vi "LP Optimal FIR Filter.vi"(1 "Band Parameters":T1(array[cluster]), 2 "# of taps":i32) -> (0 "h new":dbl[](array[numeric]))   [LabVIEW 2023]
doc: "LP Optimal FIR Filter."
uses:
  <vilib>/Analysis/1siggen.llb/Ramp Pattern by Samples.vi
  <vilib>/Analysis/NI_AALBase.lvlib
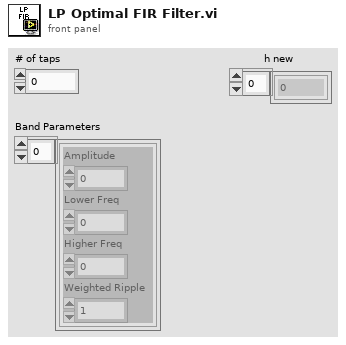
[diagram p1: front panel]
types:
  T1 = cluster{"Amplitude":dbl, "Lower Freq":dbl, "Higher Freq":dbl, "Weighted Ripple":dbl}[]
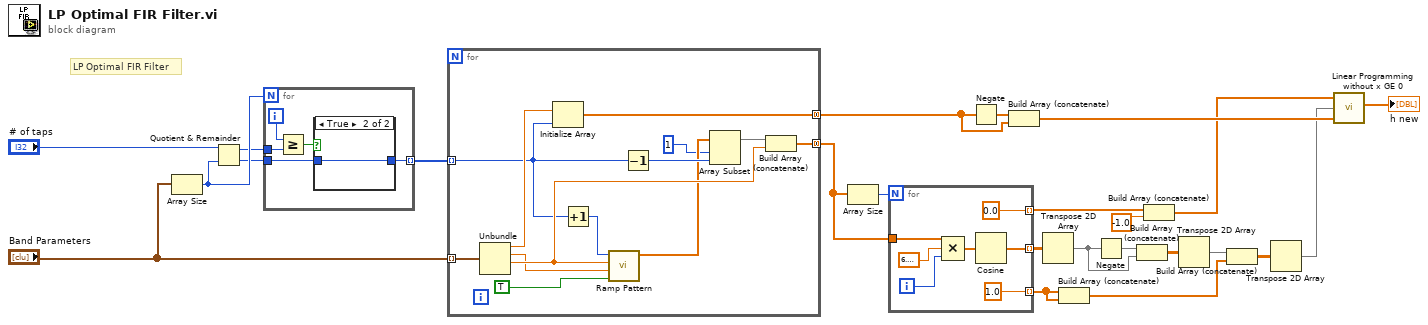
[diagram p0: block diagram]
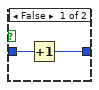
[diagram p2: hidden frame]
diagram:
  # "LP Optimal FIR Filter"
  n1 = Array Size(array="Band Parameters") -> (size(s)=w24:i32)
  n2 = Quotient & Remainder(x="# of taps", y=w24) -> (x-y*floor(x/y)=w23:i32, floor(x/y)=w22:i32)
  n3 = for {
    N: w24 -> [_]
    tunnel: w23 -> [w29]
    tunnel: w22 -> [w26]
    tunnel: [w25] -> w21 mode=indexing
    i -> [w28]
    n4 = Greater Or Equal?(x=w28, y=w29) -> (x >= y?=w27:bool)
    n5 = case shown="True" w27 {
      tunnel: w26 -> [w31 w32]
      tunnel: [w30 w32] -> w25
      frame False {
        n6 = Increment(x=w31) -> (x+1=w30:i32)
      }
      frame True {
      }
    }
  }
  n7 = for {
    tunnel: "Band Parameters" -> [w45] mode=indexing
    tunnel: w21 -> [w36] mode=indexing
    tunnel: [w35] -> w4 mode=concatenating
    tunnel: [w38] -> w2 mode=concatenating
    n8 = Unbundle(w45) -> ("Amplitude"=w37:dbl, "Lower Freq"=w34:dbl, "Higher Freq"=w41:dbl)  [unwired: 1 out]
    n9 = Initialize Array(w37, w36) -> (w35:dbl[])
    n10 = Increment(x=w36) -> (x+1=w42:i32)
    n11 = call-poly <vilib>:"Ramp Pattern.vi"("exclude end?"=TRUE, "start"=w34, "end"=w41, "samples"=w42) -> ("Ramp Pattern"=w39:dbl[])  [unwired: 6 in, 1 out]
    n12 = Decrement(x=w36) -> (x-1=w44:i32)
    n13 = Array Subset(array=w39, index=1, length=w44) -> (w43:dbl[])
    n14 = Build Array (concatenate)(w43, w41) -> (w38:dbl[])
  }
  n15 = Array Size(array=w2) -> (size(s)=w1:i32)
  n16 = for {
    N: w1 -> [_]
    tunnel: w2 -> [w52]
    tunnel: [w51] -> w8 mode=indexing
    tunnel: [1.0] -> w19 mode=indexing
    tunnel: [0.0] -> w12 mode=indexing
    i -> [w47]
    n17 = Compound Arithmetic op=MULTIPLY(w52, 6.283185307179586, w47) -> (w46:dbl[])
    n18 = Cosine(x=w46) -> (cos(x)=w51:dbl[])
  }
  n19 = Negate(x=w4) -> (-x=w18:dbl[])
  n20 = Build Array (concatenate)(w18, w4) -> (w13:dbl[])
  n21 = Transpose 2D Array(2D array=w8) -> (transposed array=w7:dbl[][])
  n22 = Build Array (concatenate)(w19, w19) -> (w14:dbl[])
  n23 = Negate(x=w7) -> (-x=w20:dbl[][])
  n24 = Build Array (concatenate)(w20, w7) -> (w15:dbl[][])
  n25 = Build Array (concatenate)(w12, -1.0) -> (w11:dbl[])
  n26 = Transpose 2D Array(2D array=w15) -> (transposed array=w17:dbl[][])
  n27 = Build Array (concatenate)(w17, w14) -> (w16:dbl[][])
  n28 = Transpose 2D Array(2D array=w16) -> (transposed array=w10:dbl[][])
  n29 = call "Linear Programming without x GE 0.vi"("C"=w11, "M"=w10, "B"=w13) -> ("X"=→"h new":dbl[])  [unwired: 3 out]
